vi "Execute Reader.vi"(8 "error in (no error)":errorcluster, 10 "Query?":bool, 11 ".NET Refnum in":refnum<k24>) -> (0 "error out":errorcluster, 2 "Data":string[][](array[string]), 3 ".NET Refnum out":refnum<k24>)   [LabVIEW 2017, in "VIs to Interface LabVIEW and MySQL dotNET Connector.lvlib"]
doc: "This VI executes a command and returns data if Query? is True and the command has return data."
uses:
  VIs to Interface LabVIEW and MySQL dotNET Connector.lvlib
  MySql.Data
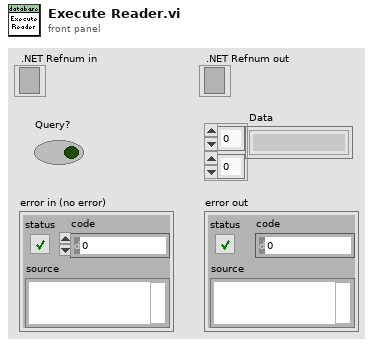
[diagram p1: front panel]
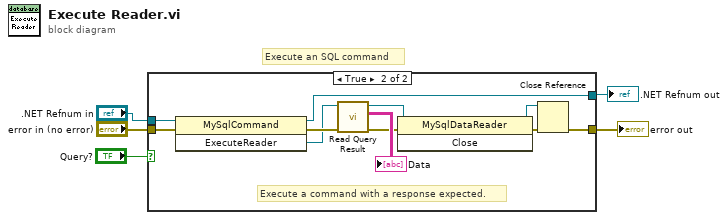
[diagram p0: block diagram]
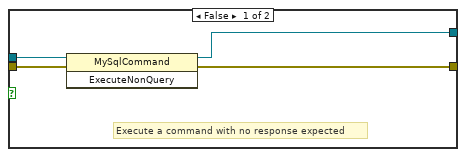
[diagram p2: hidden frame]
diagram:
  # "Execute an SQL command"
  n1 = case shown="True" "Query?" {
    tunnel: [w6 w14] -> w1
    tunnel: [w7 w19] -> w5
    tunnel: ".NET Refnum in" -> [w8 w16]
    tunnel: "error in (no error)" -> [w9 w15]
    frame False {
      # "Execute a command with no response expected"
      n2 = invoke class="MySqlCommand" method="ExecuteNonQuery"(reference=w8, error in=w9) -> (reference out=w7:refnum<k24>, error out=w6:errorcluster)  [unwired: 1 in, 1 out]
    }
    frame True {
      # "Execute a command with a response expected."
      n3 = invoke class="MySqlCommand" method="ExecuteReader"(reference=w16, error in=w15) -> (reference out=w19:refnum<k24>, error out=w18:errorcluster, "ExecuteReader"=w17:refnum<k24>)  [unwired: 1 in]
      n4 = call "Read Query Result.vi"("error in (no error)"=w18, ".NET Refnum in"=w17) -> ("error out"=w13:errorcluster, "Data"=→"Data":string[][], ".NET Refnum out"=w11:refnum<k24>)  [unwired: 7 in]
      n5 = invoke class="MySqlDataReader" method="Close"(reference=w11, error in=w13) -> (reference out=w10:refnum<k24>, error out=w12:errorcluster)  [unwired: 1 in, 1 out]
      n6 = Close Reference(reference=w10, error in (no error)=w12) -> (error out=w14:errorcluster)
    }
  }
  "error out" <- w1
  ".NET Refnum out" <- w5
